vi "motor.vi"() -> ()   [LabVIEW 2018]
uses:
  MotorController/#include/Global textParse.vi
  <instrlib>/RIGOL DS1000 Series/RIGOL DS1000 Series.lvlib
panel:
  out "Imotor Measure":dbl
  out "Imotor":bool
  in  "E-Stop":bool
  out "FoldBack":bool
  out "FoldBack Measure":dbl
  out "Current Limit Measure":dbl
  out "Current Limit":bool
  out "IRComp Measure":dbl
  out "IRComp":bool
  out "Pot high":bool
  out "Pot high Measure":dbl
  out "Pot low":bool
  out "Pot low Measure":dbl
  out "Pot mid":bool
  out "Pot mid Measure":dbl
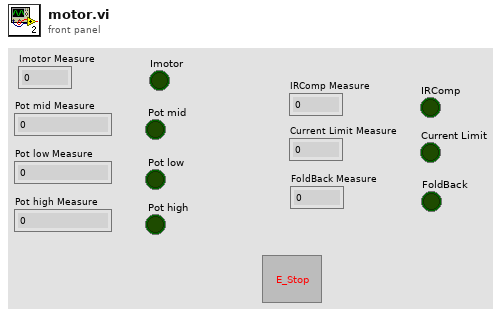
[diagram p1: front panel]
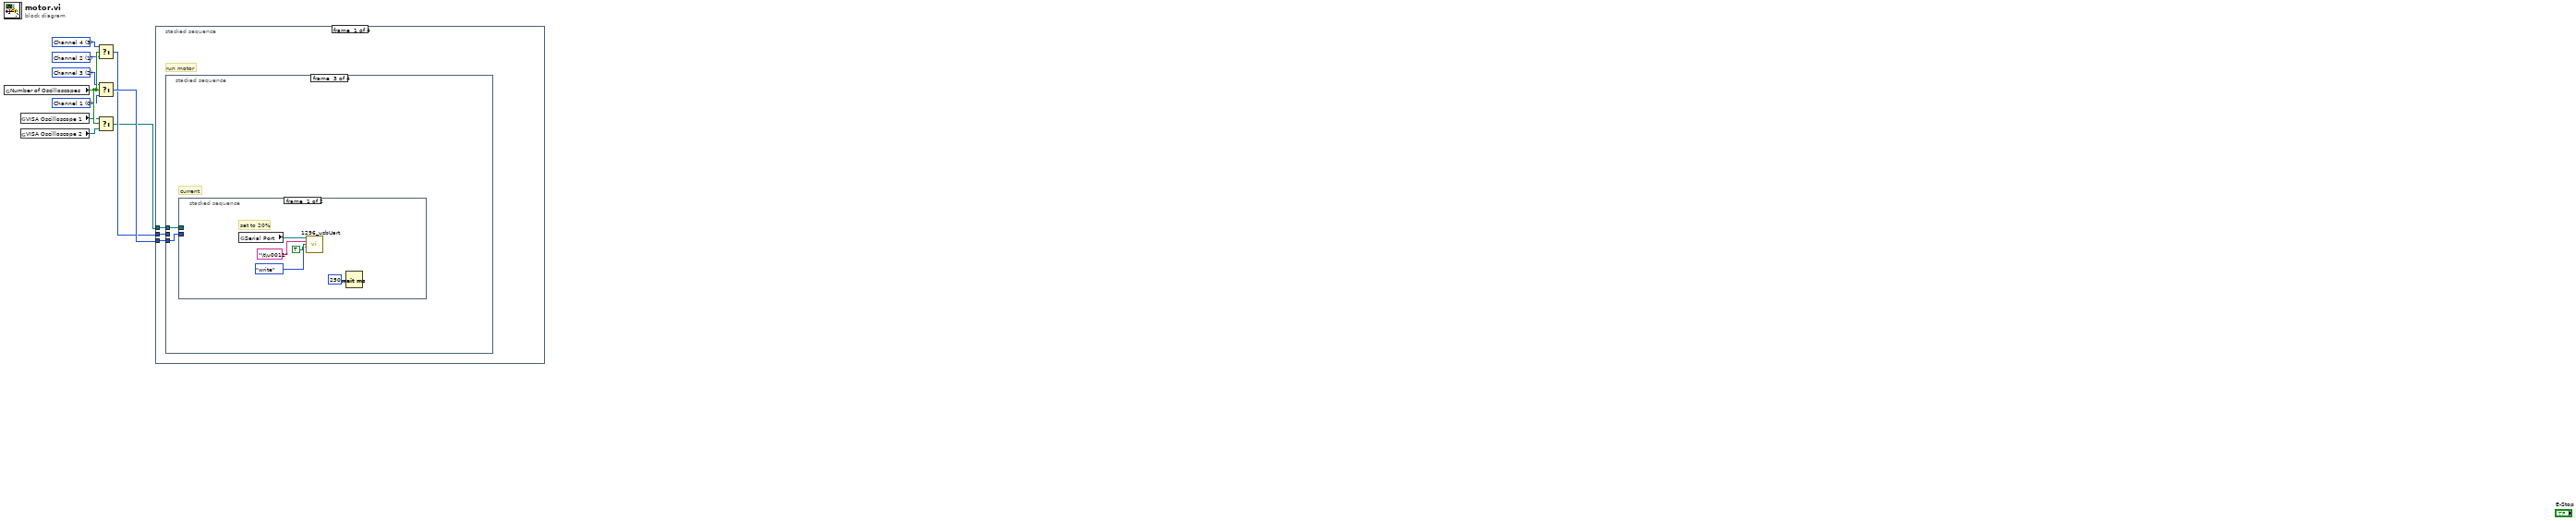
[diagram p0: block diagram]
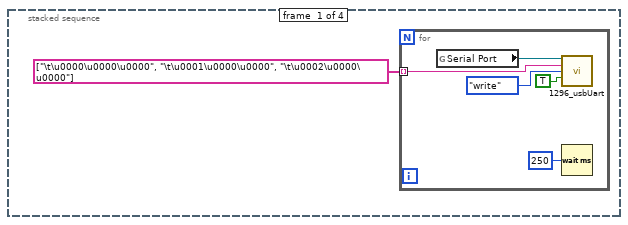
[diagram p2: hidden frame]
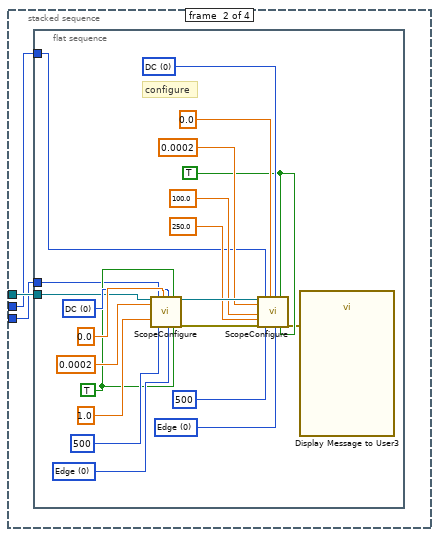
[diagram p3: hidden frame]
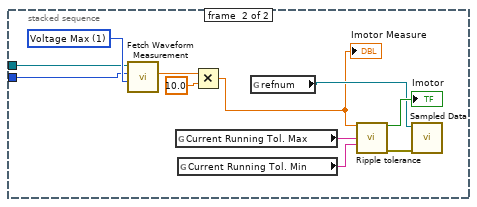
[diagram p4: hidden frame]
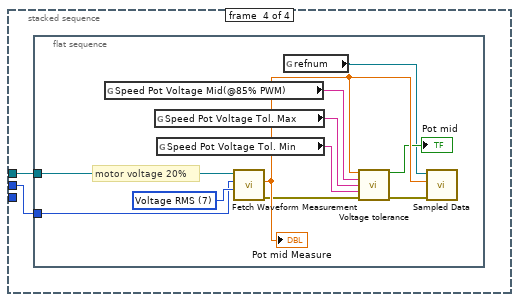
[diagram p5: hidden frame]
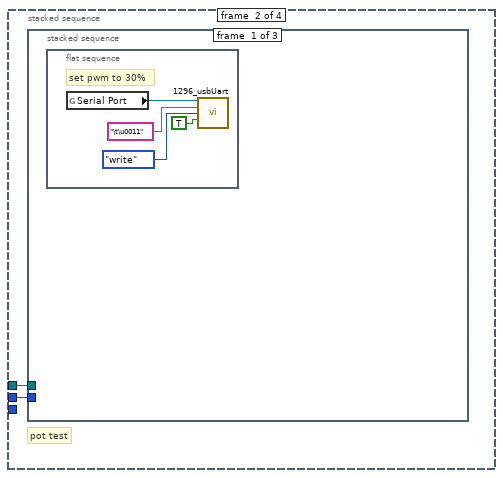
[diagram p6: hidden frame]
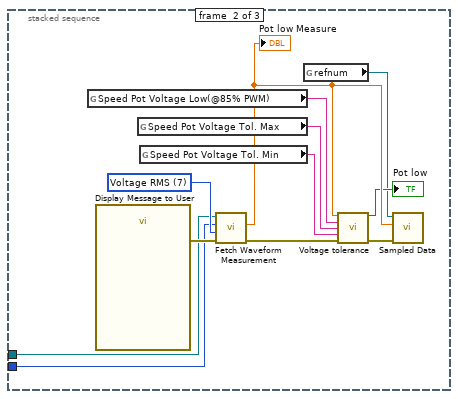
[diagram p7: hidden frame]
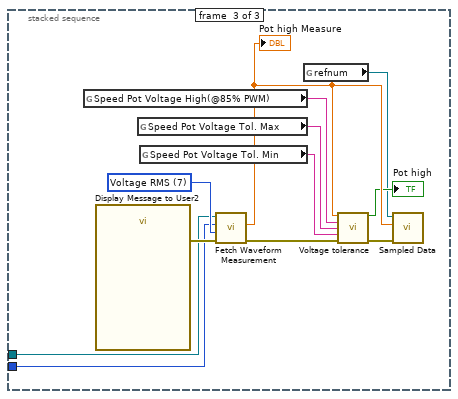
[diagram p8: hidden frame]
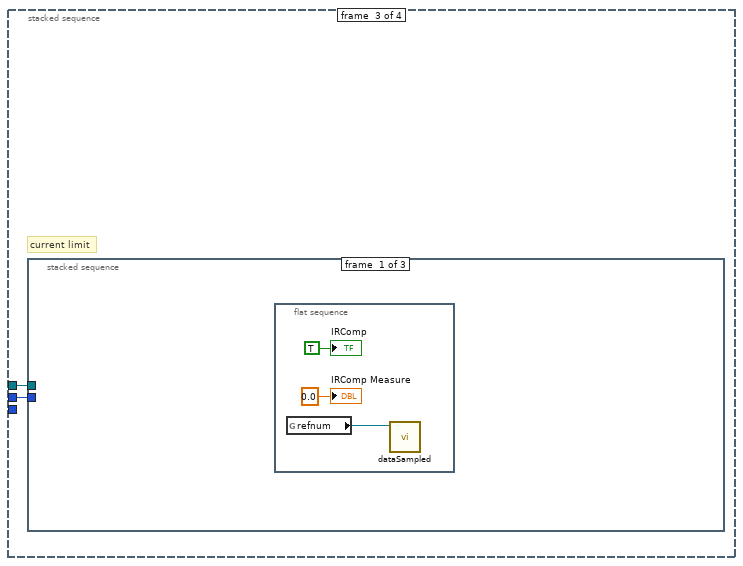
[diagram p9: hidden frame]
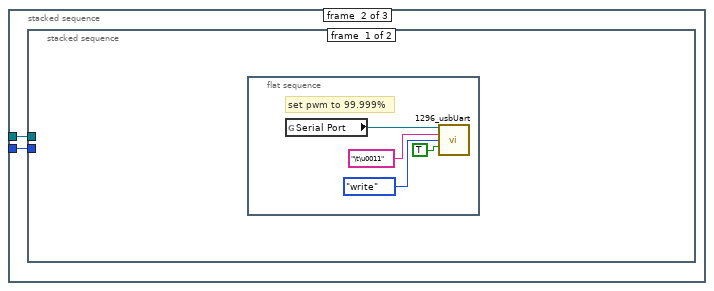
[diagram p10: hidden frame]
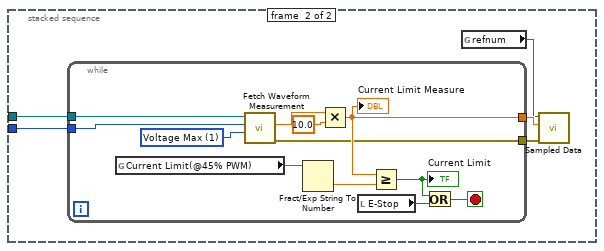
[diagram p11: hidden frame]
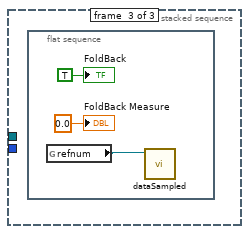
[diagram p12: hidden frame]
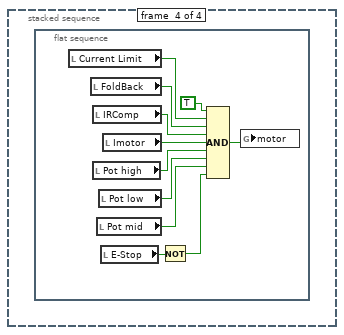
[diagram p13: hidden frame]
diagram:
  w7 = u16 0 items=["Channel 1", "Channel 2", "Channel 3", "Channel 4"] ("Source (0: Channel 1)")
  w6 = u16 2 items=["Channel 1", "Channel 2", "Channel 3", "Channel 4"] ("Source (0: Channel 1)")
  w5 = u16 1 items=["Channel 1", "Channel 2", "Channel 3", "Channel 4"] ("Source (0: Channel 1)")
  w4 = u16 3 items=["Channel 1", "Channel 2", "Channel 3", "Channel 4"] ("Source (0: Channel 1)")
  n1 = global read "Global textParse.vi" "Number of Oscilloscopes"() -> (w10:bool)
  n2 = global read "Global textParse.vi" "VISA Oscilloscope 1"() -> (w8:refnum<visa-resource-name>)
  n3 = global read "Global textParse.vi" "VISA Oscilloscope 2"() -> (w9:refnum<visa-resource-name>)
  n4 = Select(t=w4, s=w10, f=w5) -> (s? t:f=w2:u16)
  n5 = Select(t=w6, s=w10, f=w7) -> (s? t:f=w3:u16)
  n6 = Select(t=w8, s=w10, f=w9) -> (s? t:f=w1:refnum<visa-resource-name>)
  n7 = stacked-sequence {
    tunnel: w1 -> [w13 w76 w105 _]
    tunnel: w2 -> [w12 w75 w106 _]
    tunnel: w3 -> [w11 _ _ _]
    frame #0 {
      # "run motor"
      n8 = stacked-sequence {
        tunnel: w13 -> [_ w22 w45 w63]
        tunnel: w12 -> [_ w21 _ w62]
        tunnel: w11 -> [_ w20 w44 _]
        frame #0 {
          n9 = for {
            tunnel: string[] ["\t\u0000\u0000\u0000", "\t\u0001\u0000\u0000", "\t\u0002\u0000\u0000"] -> [w16] mode=indexing
            n10 = global read "Global textParse.vi" "Serial Port"() -> (w19:refnum<visa-resource-name>)
            n11 = call "1296_usbUart.vi"("VISA resource name"=w19, "command"=w16, "r/w"=enum16{"read", "write"}."write", "resetValues"=TRUE) -> ()  [unwired: 8 in, 4 out]
            n12 = Wait (ms)(milliseconds to wait=u32 250) -> ()  [unwired: 1 out]
          }
        }
        frame #1 {
          n13 = flat-sequence {
            tunnel: w22 -> [w25]
            tunnel: w21 -> [w24]
            tunnel: w20 -> [w23]
            frame #0 {
              w31 = u16 0 items=["DC", "AC", "Ground"] ("Vertical Coupling (0: DC)")
              w29 = TRUE
              w30 = u16 0 items=["Edge", "Pulse", "Video", "Pattern", "Duration"] ("Trigger Type (0: Edge)")
              w38 = u16 0 items=["DC", "AC", "Ground"] ("Vertical Coupling (0: DC)")
              w36 = TRUE
              w37 = u16 0 items=["Edge", "Pulse", "Video", "Pattern", "Duration"] ("Trigger Type (0: Edge)")
              # "configure"
              n14 = call "ScopeConfigure.vi"("VISA resource name"=w25, "scaleTime"=0.0002, "scaleVoltage"=1.0, "Channel (0: Channel 1)"=w23, "Attenuation"=500, "offsetVoltage"=0.0, "Vertical Coupling (0: DC)"=w38, "Trigger Type (0: Edge)"=w37, "BW Selector"=w36, "F Selector"=w36) -> ("VISA resource name out"=w43:refnum<visa-resource-name>, "error out"=w27:errorcluster)  [unwired: 8 in]
              n15 = call "ScopeConfigure.vi"("VISA resource name"=w43, "scaleTime"=0.0002, "triggerVoltage"=100.0, "scaleVoltage"=250.0, "error in (no error)"=w27, "Channel (0: Channel 1)"=w24, "Attenuation"=500, "offsetVoltage"=0.0, "Vertical Coupling (0: DC)"=w31, "Trigger Type (0: Edge)"=w30, "BW Selector"=w29, "F Selector"=w29) -> ("error out"=w26:errorcluster)  [unwired: 6 in, 1 out]
              n16 = call "Display Message to User3"("error in (no error)"=w26) -> ()  [unwired: 9 in, 2 out]
            }
          }
        }
        frame #2 {
          # "current"
          n17 = stacked-sequence {
            tunnel: w45 -> [_ w58]
            tunnel: w44 -> [_ w57]
            frame #0 {
              # "set to 20%"
              n18 = global read "Global textParse.vi" "Serial Port"() -> (w50:refnum<visa-resource-name>)
              n19 = call "1296_usbUart.vi"("VISA resource name"=w50, "command"="\t\u0011", "r/w"=enum16{"read", "write"}."write", "resetValues"=TRUE) -> ()  [unwired: 8 in, 4 out]
              n20 = Wait (ms)(milliseconds to wait=u32 250) -> ()  [unwired: 1 out]
            }
            frame #1 {
              w59 = u16 1 items=["Voltage Vpp", "Voltage Max", "Voltage Min", "Amplitude", "Voltage TOP", "Voltage Base", "Voltage Average", "Voltage RMS", "Overshoot", "Preshoot", "Frequency", "Rise Time", "Fall Time", "Period", "Positive Width", "Negative Width", "Positive Duty", "Negative Duty"] ("Measurement Function (0: Voltage Vpp)")
              n21 = call <instrlib>:"Fetch Waveform Measurement.vi"("Measurement Function (0: Voltage Vpp)"=w59, "Source (0: Channel 1)"=w57, "VISA resource name"=w58) -> ("Measured Value"=w61:dbl)  [unwired: 6 in, 2 out]
              n22 = global read "Global textParse.vi" "Current Running Tol. Max"() -> (w53:string)
              n23 = global read "Global textParse.vi" "Current Running Tol. Min"() -> (w54:string)
              n24 = Multiply(x=w61, y=10.0) -> (x*y=w51:dbl)
              "Imotor Measure" <- w51
              n25 = global read "Global textParse.vi" "refnum"() -> (w52:refnum<file>)
              n26 = call "Ripple tolerance.vi"("Data Sample"=w51, "Upper"=w53, "Lower"=w54) -> ("Boolean"=→"Imotor":bool, "error out"=w56:errorcluster)  [unwired: 11 in]
              n27 = call "Sampled Data.vi"("Error In"=w56, "refnum in"=w52) -> ()  [unwired: 8 in, 2 out]
            }
          }
        }
        frame #3 {
          n28 = flat-sequence {
            tunnel: w63 -> [w66]
            tunnel: w62 -> [w65]
            frame #0 {
              w67 = u16 7 items=["Voltage Vpp", "Voltage Max", "Voltage Min", "Amplitude", "Voltage TOP", "Voltage Base", "Voltage Average", "Voltage RMS", "Overshoot", "Preshoot", "Frequency", "Rise Time", "Fall Time", "Period", "Positive Width", "Negative Width", "Positive Duty", "Negative Duty"] ("Measurement Function (0: Voltage Vpp)")
              # "motor voltage 20%"
              n29 = global read "Global textParse.vi" "Speed Pot Voltage Mid(@85% PWM)"() -> (w68:string)
              n30 = global read "Global textParse.vi" "Speed Pot Voltage Tol. Max"() -> (w69:string)
              n31 = global read "Global textParse.vi" "Speed Pot Voltage Tol. Min"() -> (w70:string)
              n32 = call <instrlib>:"Fetch Waveform Measurement.vi"("Measurement Function (0: Voltage Vpp)"=w67, "Source (0: Channel 1)"=w65, "VISA resource name"=w66) -> ("error out"=w72:errorcluster, "Measured Value"=w74:dbl)  [unwired: 6 in, 1 out]
              "Pot mid Measure" <- w74
              n33 = global read "Global textParse.vi" "refnum"() -> (w64:refnum<file>)
              n34 = call "Voltage tolerance.vi"("Data Sample"=w74, "Spec Output"=w68, "Upper"=w69, "Lower"=w70, "error in (no error)"=w72) -> ("Boolean"=→"Pot mid":bool, "error out"=w71:errorcluster)  [unwired: 9 in]
              n35 = call "Sampled Data.vi"("Error In"=w71, "Data Sample"=w74, "refnum in"=w64) -> ()  [unwired: 7 in, 2 out]
            }
          }
        }
      }
    }
    frame #1 {
      # "pot test"
      n36 = stacked-sequence {
        tunnel: w76 -> [_ w83 w94]
        tunnel: w75 -> [_ w82 w95]
        frame #0 {
          n37 = flat-sequence {
            frame #0 {
              # "set pwm to 30%"
              n38 = global read "Global textParse.vi" "Serial Port"() -> (w80:refnum<visa-resource-name>)
              n39 = call "1296_usbUart.vi"("VISA resource name"=w80, "command"="\t\u0011", "r/w"=enum16{"read", "write"}."write", "resetValues"=TRUE) -> ()  [unwired: 8 in, 4 out]
            }
          }
        }
        frame #1 {
          w84 = u16 7 items=["Voltage Vpp", "Voltage Max", "Voltage Min", "Amplitude", "Voltage TOP", "Voltage Base", "Voltage Average", "Voltage RMS", "Overshoot", "Preshoot", "Frequency", "Rise Time", "Fall Time", "Period", "Positive Width", "Negative Width", "Positive Duty", "Negative Duty"] ("Measurement Function (0: Voltage Vpp)")
          n40 = global read "Global textParse.vi" "Speed Pot Voltage Low(@85% PWM)"() -> (w85:string)
          n41 = call "Display Message to User"() -> ("error out"=w92:errorcluster)  [unwired: 10 in, 1 out]
          n42 = global read "Global textParse.vi" "Speed Pot Voltage Tol. Max"() -> (w86:string)
          n43 = global read "Global textParse.vi" "Speed Pot Voltage Tol. Min"() -> (w87:string)
          n44 = call <instrlib>:"Fetch Waveform Measurement.vi"("error in (no error)"=w92, "Measurement Function (0: Voltage Vpp)"=w84, "Source (0: Channel 1)"=w82, "VISA resource name"=w83) -> ("error out"=w90:errorcluster, "Measured Value"=w91:dbl)  [unwired: 5 in, 1 out]
          "Pot low Measure" <- w91
          n45 = global read "Global textParse.vi" "refnum"() -> (w81:refnum<file>)
          n46 = call "Voltage tolerance.vi"("Data Sample"=w91, "Spec Output"=w85, "Upper"=w86, "Lower"=w87, "error in (no error)"=w90) -> ("Boolean"=→"Pot low":bool, "error out"=w88:errorcluster)  [unwired: 9 in]
          n47 = call "Sampled Data.vi"("Error In"=w88, "Data Sample"=w91, "refnum in"=w81) -> ()  [unwired: 7 in, 2 out]
        }
        frame #2 {
          w96 = u16 7 items=["Voltage Vpp", "Voltage Max", "Voltage Min", "Amplitude", "Voltage TOP", "Voltage Base", "Voltage Average", "Voltage RMS", "Overshoot", "Preshoot", "Frequency", "Rise Time", "Fall Time", "Period", "Positive Width", "Negative Width", "Positive Duty", "Negative Duty"] ("Measurement Function (0: Voltage Vpp)")
          n48 = global read "Global textParse.vi" "Speed Pot Voltage High(@85% PWM)"() -> (w101:string)
          n49 = call "Display Message to User2"() -> ("error out"=w104:errorcluster)  [unwired: 10 in, 1 out]
          n50 = global read "Global textParse.vi" "Speed Pot Voltage Tol. Max"() -> (w100:string)
          n51 = global read "Global textParse.vi" "Speed Pot Voltage Tol. Min"() -> (w99:string)
          n52 = call <instrlib>:"Fetch Waveform Measurement.vi"("error in (no error)"=w104, "Measurement Function (0: Voltage Vpp)"=w96, "Source (0: Channel 1)"=w95, "VISA resource name"=w94) -> ("error out"=w102:errorcluster, "Measured Value"=w103:dbl)  [unwired: 5 in, 1 out]
          "Pot high Measure" <- w103
          n53 = global read "Global textParse.vi" "refnum"() -> (w93:refnum<file>)
          n54 = call "Voltage tolerance.vi"("Data Sample"=w103, "Spec Output"=w101, "Upper"=w100, "Lower"=w99, "error in (no error)"=w102) -> ("Boolean"=→"Pot high":bool, "error out"=w98:errorcluster)  [unwired: 9 in]
          n55 = call "Sampled Data.vi"("Error In"=w98, "Data Sample"=w103, "refnum in"=w93) -> ()  [unwired: 7 in, 2 out]
        }
      }
    }
    frame #2 {
      # "current limit"
      n56 = stacked-sequence {
        tunnel: w105 -> [_ w111 _]
        tunnel: w106 -> [_ w110 _]
        frame #0 {
          n57 = flat-sequence {
            frame #0 {
              n58 = global read "Global textParse.vi" "refnum"() -> (w107:refnum<file>)
              n59 = call "dataSampled.vi"("refnum in"=w107) -> ()  [unwired: 9 in, 2 out]
              "IRComp Measure" <- 0.0 ("IRComp Measeure")
              "IRComp" <- TRUE ("IRComp")
            }
          }
        }
        frame #1 {
          n60 = stacked-sequence {
            tunnel: w111 -> [_ w117]
            tunnel: w110 -> [_ w116]
            frame #0 {
              n61 = flat-sequence {
                frame #0 {
                  # "set pwm to 99.999%"
                  n62 = global read "Global textParse.vi" "Serial Port"() -> (w115:refnum<visa-resource-name>)
                  n63 = call "1296_usbUart.vi"("VISA resource name"=w115, "command"="\t\u0011", "r/w"=enum16{"read", "write"}."write", "resetValues"=TRUE) -> ()  [unwired: 8 in, 4 out]
                }
              }
            }
            frame #1 {
              n64 = while {
                tunnel: w117 -> [w127]
                tunnel: w116 -> [w126]
                tunnel: [w125] -> w119
                tunnel: [w121] -> w120
                stop <- w124 stop-if-true
                w130 = u16 1 items=["Voltage Vpp", "Voltage Max", "Voltage Min", "Amplitude", "Voltage TOP", "Voltage Base", "Voltage Average", "Voltage RMS", "Overshoot", "Preshoot", "Frequency", "Rise Time", "Fall Time", "Period", "Positive Width", "Negative Width", "Positive Duty", "Negative Duty"] ("Measurement Function (0: Voltage Vpp)")
                n65 = global read "Global textParse.vi" "Current Limit(@45% PWM)"() -> (w128:string)
                n66 = call <instrlib>:"Fetch Waveform Measurement.vi"("Measurement Function (0: Voltage Vpp)"=w130, "Source (0: Channel 1)"=w126, "VISA resource name"=w127) -> ("error out"=w121:errorcluster, "Measured Value"=w132:dbl)  [unwired: 6 in, 1 out]
                n67 = Fract/Exp String To Number(string=w128) -> (number=w129:dbl)  [unwired: 3 in, 1 out]
                n68 = Multiply(x=w132, y=10.0) -> (x*y=w125:dbl)
                "Current Limit Measure" <- w125
                n69 = local read "E-Stop"() -> (w122:bool)
                n70 = Greater Or Equal?(x=w125, y=w129) -> (x >= y?=w123:bool)
                "Current Limit" <- w123
                n71 = Or(x=w123, y=w122) -> (x .or. y?=w124:bool)
              }
              n72 = global read "Global textParse.vi" "refnum"() -> (w118:refnum<file>)
              n73 = call "Sampled Data.vi"("Error In"=w120, "Data Sample"=w119, "refnum in"=w118) -> ()  [unwired: 7 in, 2 out]
            }
          }
        }
        frame #2 {
          n74 = flat-sequence {
            frame #0 {
              n75 = global read "Global textParse.vi" "refnum"() -> (w133:refnum<file>)
              n76 = call "dataSampled.vi"("refnum in"=w133) -> ()  [unwired: 9 in, 2 out]
              "FoldBack" <- TRUE ("FoldBack")
              "FoldBack Measure" <- 0.0 ("FoldBack Measure")
            }
          }
        }
      }
    }
    frame #3 {
      n77 = flat-sequence {
        frame #0 {
          n78 = local read "Current Limit"() -> (w144:bool)
          n79 = local read "FoldBack"() -> (w143:bool)
          n80 = local read "IRComp"() -> (w142:bool)
          n81 = local read "Pot high"() -> (w141:bool)
          n82 = local read "Pot mid"() -> (w139:bool)
          n83 = local read "Pot low"() -> (w140:bool)
          n84 = local read "E-Stop"() -> (w138:bool)
          n85 = local read "Imotor"() -> (w136:bool)
          n86 = Not(x=w138) -> (.not. x?=w137:bool)
          n87 = Compound Arithmetic op=AND(TRUE ("value"), w144, w143, w142, w136, w141, w140, w139, w137) -> (w146:bool)
          n88 = global write "Global textParse.vi" "motor"(w146) -> ()
        }
      }
    }
  }
